vi "WPI_PWMSafetyCheck.vi"(0 "PWMDeviceRef":T1={"DeviceStatus"={"status"=FALSE, "code"=0, "source"=""}, "PWM Channel"=enum."PWM 1"}, 5 "menu":T3, 7 "VI Refnum":refnum<vi>, 9 "timeout (ms)":u32=100, 11 "error in (no error)":errorcluster) -> (15 "error out":errorcluster)   [LabVIEW 2017]
doc: "This subVI holds an array of DevRefs, timeout values, and latest update times. These values can be added, updated, tested, and removed.\n\nThis gets called by Open to add a set of values. It gets called by Drive to update the 'last update value'. It gets called by Close to remove a set of values.\n\nIt also gets called by Safety Test via the SafetyCheckEngine that runs as a background task called by the Start Communication loop to test all sets of values for a timeout condition.\n\nThis software is licensed. Open the labview\\readme\\WPI Robotics Library Open Source License.txt file for more information."
uses:
  <vilib>/Rock Robotics/WPI/SafetyOutput/WPI_SafetyOutputCheckMenu.ctl
  <vilib>/Rock Robotics/WPI/PWM/WPI_PWMDeviceRef.ctl
  <vilib>/Rock Robotics/SystemInterfaces/DIO/FPGA_DIOPWMChannel.ctl
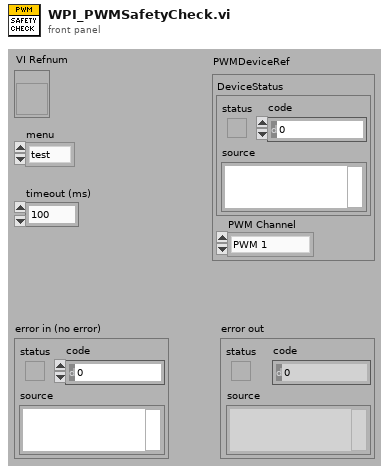
[diagram p1: front panel]
types:
  T1 = typedef "WPI_PWMDeviceRef.ctl" = cluster{"DeviceStatus":errorcluster, "PWM Channel":T2}
  T2 = typedef "FPGA_DIOPWMChannel.ctl" = enum8{"PWM 0", "PWM 1", "PWM 2", "PWM 3", "PWM 4", "PWM 5", "PWM 6", "PWM 7", "PWM 8", "PWM 9", "PWM MXP 0", "PWM MXP 1", "PWM MXP 2", "PWM MXP 3", "PWM MXP 4", "PWM MXP 5", "PWM MXP 6", "PWM MXP 7", "PWM MXP 8", "PWM MXP 9", "Invalid"}
  T3 = typedef "WPI_SafetyOutputCheckMenu.ctl" = enum16{"test", "add", "remove", "update"}
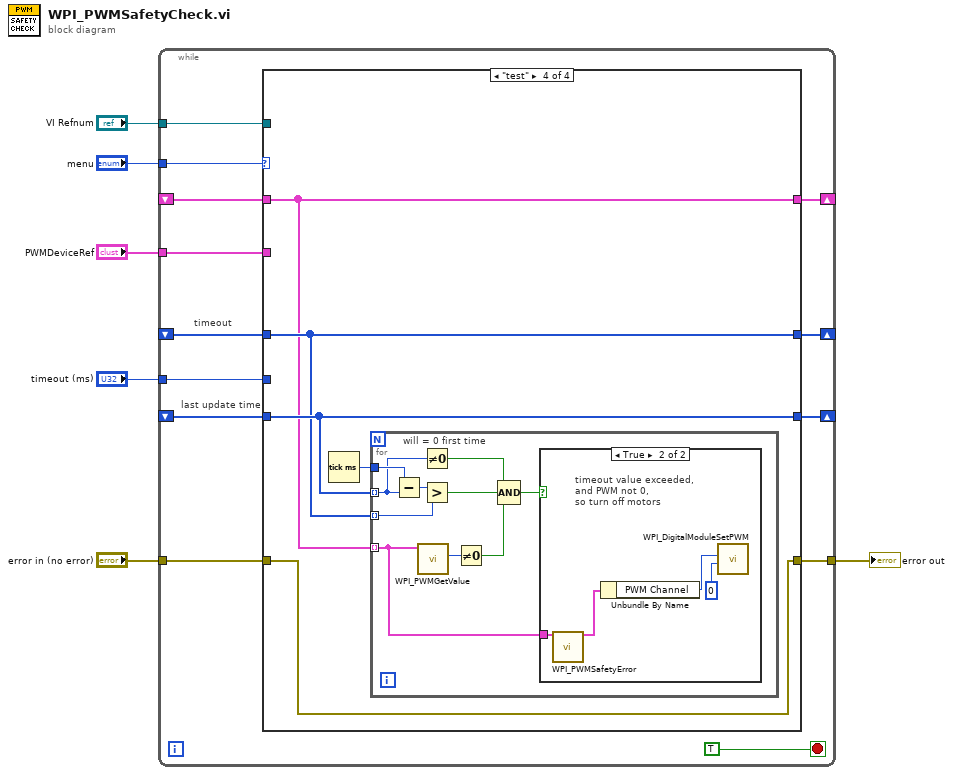
[diagram p0: block diagram]
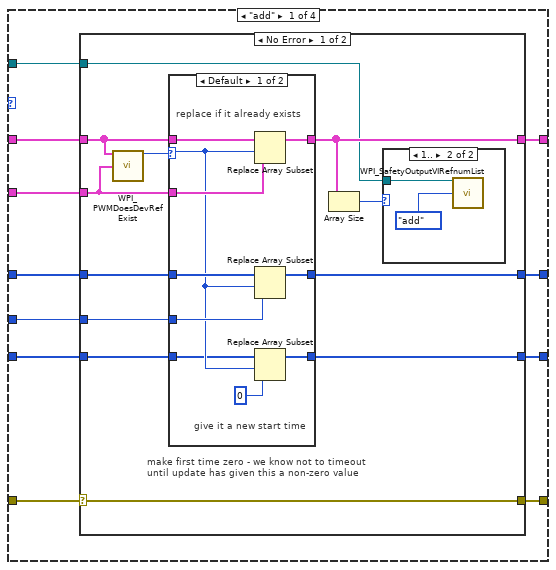
[diagram p2: hidden frame]
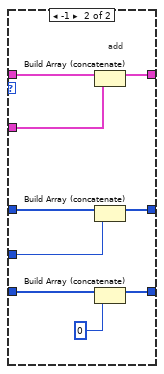
[diagram p4: hidden frame]
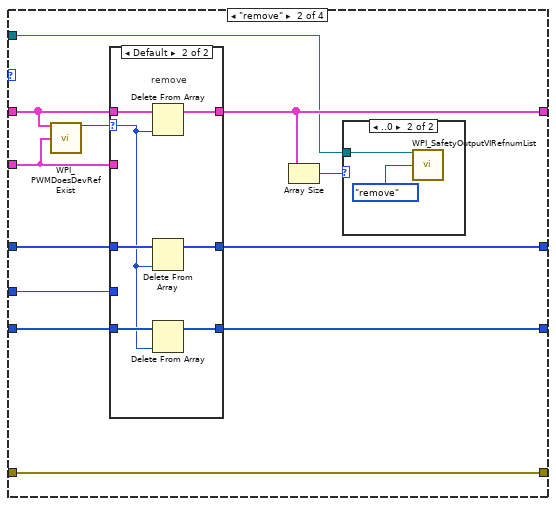
[diagram p6: hidden frame]
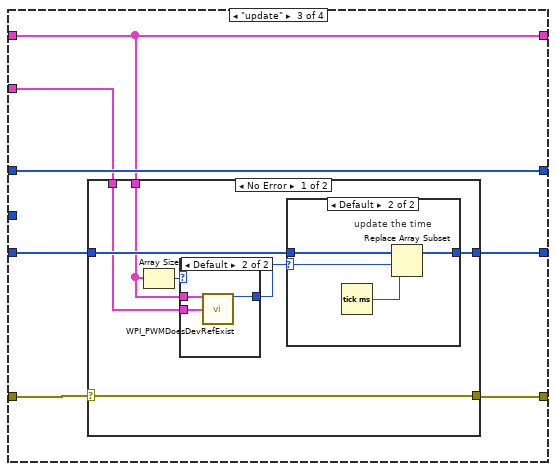
[diagram p9: hidden frame]
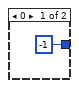
[diagram p10: hidden frame]
diagram:
  n1 = while {
    tunnel: "menu" -> [w18]
    shift-right: [w17] -> _
    shift-left: _ -> [w13]
    tunnel: "PWMDeviceRef" -> [w12]
    shift-right: [w14] -> _
    shift-left: _ -> [w16]
    tunnel: "timeout (ms)" -> [w15]
    shift-right: [w10] -> _
    shift-left: _ -> [w11]
    tunnel: "VI Refnum" -> [w9]
    tunnel: "error in (no error)" -> [w8]
    tunnel: [w7] -> w1
    stop <- TRUE stop-if-true
    # "last update time"
    # "timeout"
    n2 = case shown="\"test\"" w18 {
      tunnel: w13 -> [w30 w69 w93 w118]
      tunnel: [w23 w73 w93 w118] -> w17
      tunnel: w12 -> [w29 w68 w92 _]
      tunnel: w16 -> [w28 w79 w98 w119]
      tunnel: w15 -> [w27 w78 _ _]
      tunnel: [w26 w77 w98 w119] -> w14
      tunnel: w11 -> [w25 w76 w97 w120]
      tunnel: [w24 w75 w96 w120] -> w10
      tunnel: w9 -> [w22 w72 _ _]
      tunnel: w8 -> [w21 w71 w95 w117]
      tunnel: [w20 w71 w94 w117] -> w7
      frame "add" {
        n3 = case shown="No Error" w21 {
          selector: w21 -> [w34 w67]
          tunnel: w30 -> [w33 w66]
          tunnel: w29 -> [w32 _]
          tunnel: w28 -> [w42 w65]
          tunnel: w27 -> [w41 _]
          tunnel: [w40 w65] -> w26
          tunnel: w25 -> [w39 w64]
          tunnel: [w38 w64] -> w24
          tunnel: [w37 w66] -> w23
          tunnel: w22 -> [w36 _]
          tunnel: [w34 w67] -> w20
          frame No Error {
            # "make first time zero - we know not to timeout until update has given this a non-zero value"
            n4 = call <vilib>:"WPI_PWMDoesDevRefExist.vi"("PWMDeviceRefArray"=w33, "PWMDeviceRef"=w32) -> ("index"=w31:i32)  [unwired: 13 out]
            n5 = case shown="Default" w31 {
              selector: w31 -> [w47 _]
              tunnel: w33 -> [w54 w63]
              tunnel: [w53 w62] -> w37
              tunnel: w32 -> [w52 w61]
              tunnel: w42 -> [w51 w60]
              tunnel: w41 -> [w49 w59]
              tunnel: [w50 w58] -> w40
              tunnel: w39 -> [w46 w57]
              tunnel: [w45 w56] -> w38
              frame Default {
                # "give it a new start time"
                # "replace if it already exists"
                n6 = Replace Array Subset(array=w54, new element=w52, index=w47) -> (w53:T1[])
                n7 = Replace Array Subset(array=w51, new element=w49, index=w47) -> (w50:u32[])
                n8 = Replace Array Subset(array=w46, new element=u32 0 ("millisecond timer value"), index=w47) -> (w45:u32[])
              }
              frame -1 {
                # "add"
                n9 = Build Array (concatenate)(w63, w61) -> (w62:T1[])
                n10 = Build Array (concatenate)(w60, w59) -> (w58:u32[])
                n11 = Build Array (concatenate)(w57, u32 0 ("millisecond timer value")) -> (w56:u32[])
              }
            }
            n12 = Array Size(array=w37) -> (size(s)=w35:i32)
            n13 = case shown="1.." w35 {
              tunnel: w36 -> [_ w43]
              frame Default {
              }
              frame 1.. {
                n14 = call <vilib>:"WPI_SafetyOutputVIRefnumList.vi"("VI Refnum"=w43, "menu"=enum16{"read", "add", "remove"}."add") -> ()  [unwired: 14 out]
              }
            }
          }
          frame Error {
            # "do not add if there is an error"
          }
        }
      }
      frame "remove" {
        n15 = call <vilib>:"WPI_PWMDoesDevRefExist.vi"("PWMDeviceRefArray"=w69, "PWMDeviceRef"=w68) -> ("index"=w70:i32)  [unwired: 13 out]
        n16 = case shown="Default" w70 {
          selector: w70 -> [_ w85]
          tunnel: w69 -> [w84 w91]
          tunnel: [w84 w88] -> w73
          tunnel: w68 -> [_ _]
          tunnel: w79 -> [w83 w90]
          tunnel: w78 -> [_ _]
          tunnel: [w83 w87] -> w77
          tunnel: w76 -> [w82 w89]
          tunnel: [w82 w86] -> w75
          frame -1 {
            # "do nothing if it does not exist"
          }
          frame Default {
            # "remove"
            n17 = Delete From Array(array=w91, index=w85) -> (array with subset deleted=w88:T1[])  [unwired: 1 in, 1 out]
            n18 = Delete From Array(array=w90, index=w85) -> (array with subset deleted=w87:u32[])  [unwired: 1 in, 1 out]
            n19 = Delete From Array(array=w89, index=w85) -> (array with subset deleted=w86:u32[])  [unwired: 1 in, 1 out]
          }
        }
        n20 = Array Size(array=w73) -> (size(s)=w74:i32)
        n21 = case shown="..0" w74 {
          tunnel: w72 -> [_ w80]
          frame Default {
          }
          frame ..0 {
            n22 = call <vilib>:"WPI_SafetyOutputVIRefnumList.vi"("VI Refnum"=w80, "menu"=enum16{"read", "add", "remove"}."remove") -> ()  [unwired: 14 out]
          }
        }
      }
      frame "update" {
        n23 = case shown="No Error" w95 {
          selector: w95 -> [w103 w116]
          tunnel: w97 -> [w105 w115]
          tunnel: [w104 w115] -> w96
          tunnel: [w103 w116] -> w94
          tunnel: w93 -> [w99 _]
          tunnel: w92 -> [w101 _]
          frame No Error {
            n24 = Array Size(array=w99) -> (size(s)=w100:i32)
            n25 = case shown="Default" w100 {
              tunnel: [-1 ("index") w109] -> w102
              tunnel: w99 -> [_ w108]
              tunnel: w101 -> [_ w107]
              frame 0 {
              }
              frame Default {
                n26 = call <vilib>:"WPI_PWMDoesDevRefExist.vi"("PWMDeviceRefArray"=w108, "PWMDeviceRef"=w107) -> ("index"=w109:i32)  [unwired: 13 out]
              }
            }
            n27 = case shown="Default" w102 {
              selector: w102 -> [_ w111]
              tunnel: w105 -> [w110 w114]
              tunnel: [w110 w113] -> w104
              frame -1 {
                # "don't replace if it doesn't exist"
              }
              frame Default {
                # "update the time"
                n28 = Tick Count (ms)() -> (millisecond timer value=w112:u32)
                n29 = Replace Array Subset(array=w114, new element=w112, index=w111) -> (w113:u32[])
              }
            }
          }
          frame Error {
            # "do not update if there is an error"
          }
        }
      }
      frame "test" {
        n30 = Tick Count (ms)() -> (millisecond timer value=w121:u32)
        n31 = for {
          tunnel: w120 -> [w127] mode=indexing
          tunnel: w121 -> [w131]
          tunnel: w119 -> [w129] mode=indexing
          tunnel: w118 -> [w124] mode=indexing
          # "will = 0 first time"
          n32 = Subtract(x=w131, y=w127) -> (x-y=w130:u32)
          n33 = call <vilib>:"WPI_PWMGetValue.vi"("PWMDeviceRef"=w124) -> ("Value"=w123:u16)  [unwired: 8 in, 2 out]
          n34 = Not Equal To 0?(x=w127) -> (x != 0?=w125:bool)
          n35 = Greater?(x=w130, y=w129) -> (0:w128:bool)
          n36 = Not Equal To 0?(x=w123) -> (x != 0?=w122:bool)
          n37 = Compound Arithmetic op=AND(w125, w128, w122) -> (w126:bool)
          n38 = case shown="True" w126 {
            tunnel: w124 -> [_ w135]
            frame False {
              # "do nothing"
            }
            frame True {
              # "timeout value exceeded,\nand PWM not 0,\nso turn off motors"
              n39 = call <vilib>:"WPI_PWMSafetyError.vi"("PWMDeviceRef"=w135) -> ("PWMDeviceRef"=w132:T1)  [unwired: 14 out]
              n40 = Unbundle By Name(w132) -> ("PWM Channel"=w134:T2)
              n41 = call <vilib>:"WPI_DigitalModuleSetPWM.vi"("Speed"=u16 0, "PWMChannel"=w134) -> ()  [unwired: 4 in, 6 out]
            }
          }
        }
      }
    }
  }
  "error out" <- w1
